vi "Queue Access FGV 2013 NIVerified.vi"() -> ()   [LabVIEW 2020]
uses:
  Controls/FGV State Command.ctl
  Controls/Message Data.ctl
  Controls/State Command.ctl
panel:
  in  "Stop Button":bool
  in  "Do Something":bool
  # "Objective: This example demonstrates how an FGV can be used to store Queue references.\nRequirements: LabVIEW Full Development System\nInstructions:\n1. Run the program.\n2. Press the \"Do Something\" button to open up a dialog box.\n3. Press the \"Stop Button\" button to exit the program"
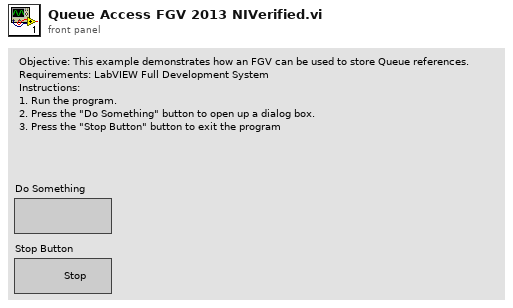
[diagram p1: front panel]
types:
  T1 = typedef "FGV State Command.ctl" = enum16{"Get", "Initialize", "Release"}
  T2 = typedef "State Command.ctl" = enum16{"Display Message", "Stop"}
  T3 = typedef "Message Data.ctl" = cluster{"State Command":T2, "Data":variant}
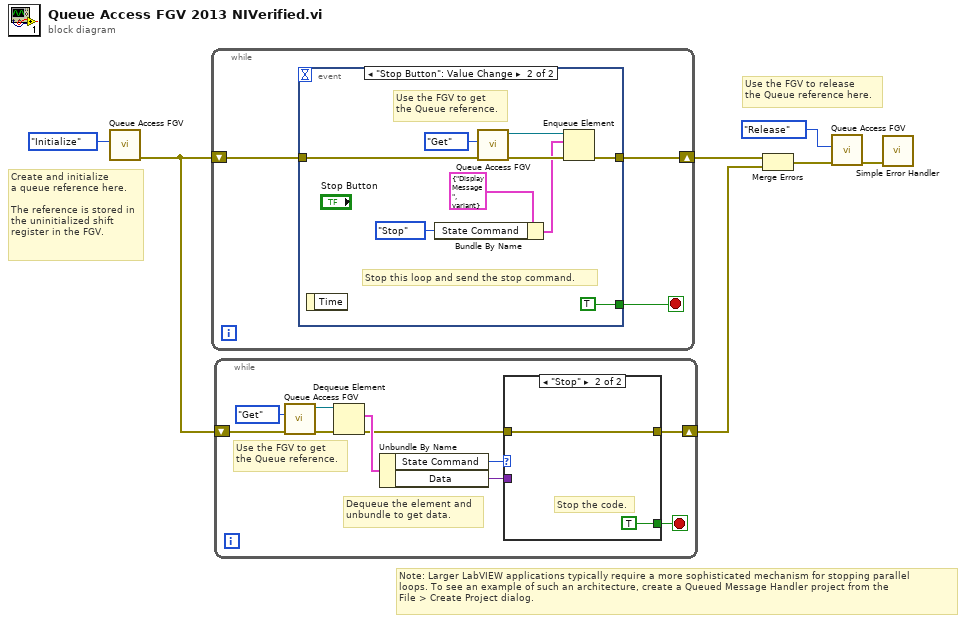
[diagram p0: block diagram]
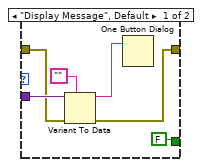
[diagram p2: hidden frame]
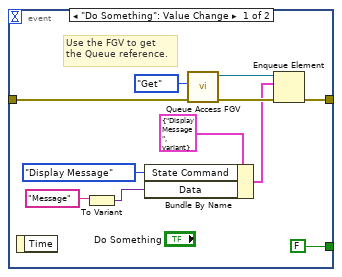
[diagram p3: hidden frame]
diagram:
  # "Use the FGV to release\nthe Queue reference here."
  # "Create and initialize\na queue reference here.\n\nThe reference is stored in\nthe uninitialized shift\nregister in the FGV."
  # "Note: Larger LabVIEW applications typically require a more sophisticated mechanism for stopping parallel\nloops. To see an example of such an architecture, create a Queued Message Handler project from the\nFile > Create Project dialog."
  n1 = call "Queue Access FGV.vi"("FGV State Command"=FGV_State_Command."Initialize") -> ("error out"=w7:errorcluster)  [unwired: 8 in, 1 out]
  n2 = while {
    shift-right: [w10] -> w6
    shift-left: w7 -> [w9]
    stop <- w8 stop-if-true
    n3 = event shown="[1] \"Stop Button\": Value Change" {
      selector: _ -> [_ _]
      dyn-events: _ -> [_ _]
      timeout: _ -> [_ _]
      tunnel: [w21 w30] -> w10
      tunnel: w9 -> [w18 w27]
      tunnel: [FALSE TRUE] -> w8
      event "Do Something": Value Change {
        # "Use the FGV to get\nthe Queue reference."
        n4 = event-data() -> ()  [unwired: 1 in, 1 out]
        n5 = To Variant(anything="Message") -> (Variant=w12:variant)
        n6 = Bundle By Name(cluster=T3 {"State Command"=enum."Display Message", "Data"=variant} ("Message Data"), "State Command"=State_Command."Display Message", "Data"=w12) -> (w15:T3)
        n7 = call "Queue Access FGV.vi"("FGV State Command"=FGV_State_Command."Get", "error in (no error)"=w18) -> ("Queue out"=w19:refnum<queue>, "error out"=w20:errorcluster)  [unwired: 7 in]
        n8 = Enqueue Element(queue=w19, element=w15, error in (no error)=w20) -> (error out=w21:errorcluster)  [unwired: 1 in, 2 out]
      }
      event "Stop Button": Value Change {
        # "Stop this loop and send the stop command."
        # "Use the FGV to get\nthe Queue reference."
        n9 = event-data() -> ()  [unwired: 1 in, 1 out]
        n10 = Bundle By Name(cluster=T3 {"State Command"=enum."Display Message", "Data"=variant} ("Message Data"), "State Command"=State_Command."Stop") -> (w24:T3)
        n11 = call "Queue Access FGV.vi"("FGV State Command"=FGV_State_Command."Get", "error in (no error)"=w27) -> ("Queue out"=w28:refnum<queue>, "error out"=w29:errorcluster)  [unwired: 7 in]
        n12 = Enqueue Element(queue=w28, element=w24, error in (no error)=w29) -> (error out=w30:errorcluster)  [unwired: 1 in, 2 out]
      }
    }
  }
  n13 = while {
    shift-right: [w33] -> w5
    shift-left: w7 -> [w37]
    stop <- w31 stop-if-true
    # "Dequeue the element and\nunbundle to get data."
    # "Use the FGV to get\nthe Queue reference."
    n14 = call "Queue Access FGV.vi"("FGV State Command"=FGV_State_Command."Get", "error in (no error)"=w37) -> ("Queue out"=w36:refnum<queue>, "error out"=w35:errorcluster)  [unwired: 7 in]
    n15 = Dequeue Element(queue=w36, error in (no error)=w35) -> (element=w40:T3, error out=w34:errorcluster)  [unwired: 1 in, 2 out]
    n16 = Unbundle By Name(w40) -> ("State Command"=w39:T2, "Data"=w38:variant)
    n17 = case shown="\"Stop\"" w39 {
      tunnel: w38 -> [w46 _]
      tunnel: w34 -> [w44 w48]
      tunnel: [w42 w48] -> w33
      tunnel: [FALSE TRUE] -> w31
      frame "Display Message", Default {
        n18 = Variant To Data(error in=w44, type="", Variant=w46) -> (data=w43:string, error out=w42:errorcluster)
        n19 = One Button Dialog(message=w43) -> ()  [unwired: 1 in, 1 out]
      }
      frame "Stop" {
        # "Stop the code."
      }
    }
  }
  n20 = Merge Errors(w6, w5) -> (w4:errorcluster)
  n21 = call "Queue Access FGV.vi"("FGV State Command"=FGV_State_Command."Release", "error in (no error)"=w4) -> ("error out"=w3:errorcluster)  [unwired: 7 in, 1 out]
  n22 = call <vilib>:"Simple Error Handler.vi"("error in (no error)"=w3) -> ()  [unwired: 4 in, 5 out]
